vi "Internet Access.vi"(10 "error in (no error)":errorcluster) -> (2 "error out":errorcluster, 3 "Connected?":bool)   [LabVIEW 2021]
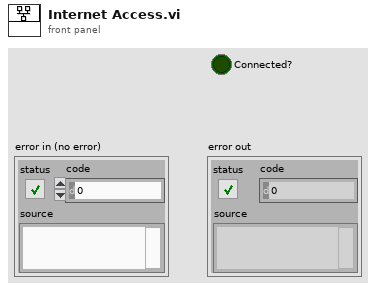
[diagram p1: front panel]
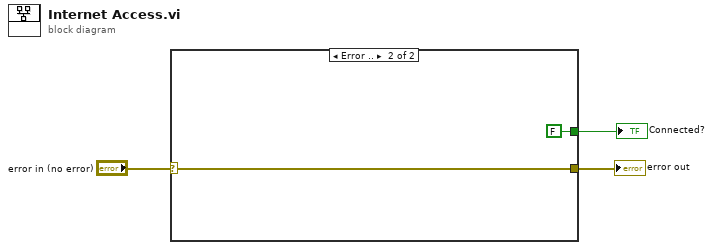
[diagram p0: block diagram]
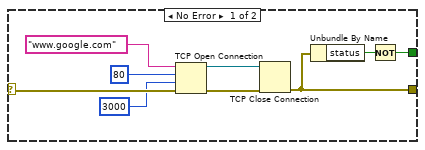
[diagram p2: hidden frame]
diagram:
  n1 = case shown="Error .." "error in (no error)" {
    selector: "error in (no error)" -> [w12 w14]
    tunnel: [w6 w14] -> w2
    tunnel: [w4 FALSE] -> w1
    frame No Error {
      n2 = TCP Open Connection(address="www.google.com", remote port or service name=u16 80, timeout ms (60000)=3000, error in (no error)=w12) -> (connection ID=w11:refnum<k5>, error out=w10:errorcluster)  [unwired: 1 in]
      n3 = TCP Close Connection(connection ID=w11, error in (no error)=w10) -> (error out=w6:errorcluster)  [unwired: 1 in, 1 out]
      n4 = Unbundle By Name(w6) -> ("status"=w5:bool)
      n5 = Not(x=w5) -> (.not. x?=w4:bool)
    }
    frame Error {
    }
  }
  "error out" <- w2
  "Connected?" <- w1
